vi "test_Error Code Channel_Overwrite File If Exists Disabled.vi"(8 "error in (no error)":errorcluster, 11 "TestCase in":refnum<class "Telemetry System Tests.lvclass">=refnum) -> (0 "error out":errorcluster, 3 "TestCase out":refnum<class "Telemetry System Tests.lvclass">)   [LabVIEW 2026, in "Telemetry System Tests.lvclass"]
uses:
  Telemetry System Tests.lvclass
  b15e678b-00b4-460c-84a3-511904b6b81c.vi
  <vilib>/NI VeriStand/Execution/Workspace/NI_VS Workspace ExecutionAPI.lvlib
  Telemetry Test Utilities/Telemetry Test Utilities.lvlib
  b783cf42-fd76-406f-8202-c013ab39f902.vi
  0f18a7fd-8127-48b0-8de3-31218f8e8d95.vi
  addb9b33-6ae5-4271-aa15-5e9a5667d6da.vi
  <vilib>/NI VeriStand/Execution/Workspace/NI VeriStand - Get Single Channel Value.vi
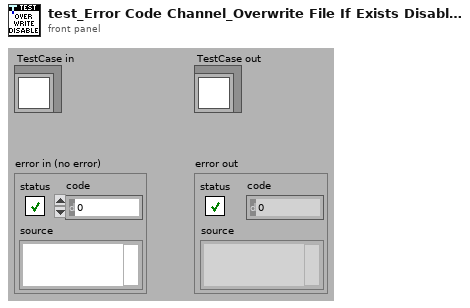
[diagram p1: front panel]
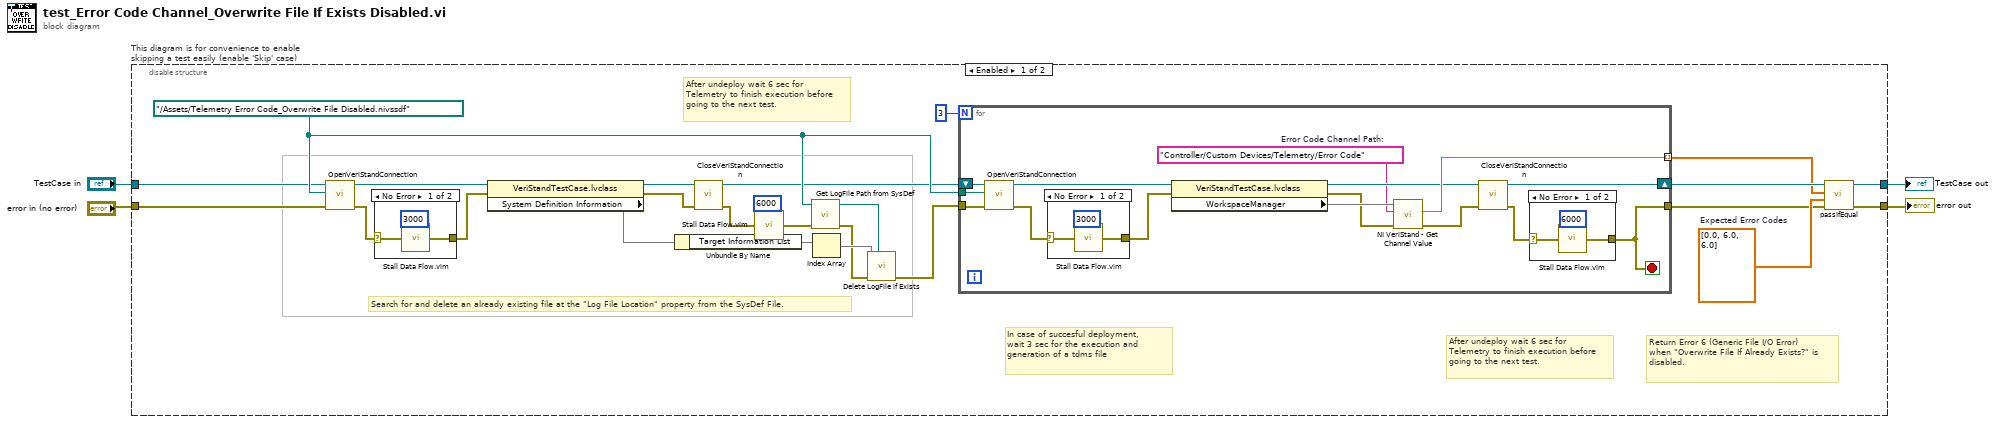
[diagram p0: block diagram]
diagram:
  n1 = disable-structure "This diagram is for convenience to enable skipping a test easily (enable 'Skip' case)" shown="Enabled" {
    disable-tunnel: "TestCase in" -> [w15 w60]
    disable-tunnel: [w23 w58] -> w1
    disable-tunnel: [w24 w59] -> w3
    disable-tunnel: "error in (no error)" -> [w18 w57]
    frame Enabled {
      w26 = dbl[] [0.0, 6.0, 6.0]  # Expected Error Codes
      w16 = path "../Assets/Telemetry Error Code_Overwrite File Disabled.nivssdf" ("System Definition File")
      # "In case of succesful deployment, wait 3 sec for the execution and generation of a tdms file"
      # "After undeploy wait 6 sec for Telemetry to finish execution before going to the next test."
      # "After undeploy wait 6 sec for Telemetry to finish execution before going to the next test."
      # "Search for and delete an already existing file at the \"Log File Location\" property from the SysDef File."
      # "Return Error 6 (Generic File I/O Error) when \"Overwrite File If Already Exists?\" is disabled."
      n2 = call-dynamic "OpenVeriStandConnection.vi"("error in (no error)"=w18, "System Definition File"=w16, "VeriStand Test Case in"=w15) -> ("error out"=w17:errorcluster, "VeriStand Test Case out"=w14:refnum<class "VeriStandTestCase.lvclass">)  [unwired: 6 in, 1 out]
      n3 = case shown="No Error" w17 {
        selector: w17 -> [w32 w33]
        tunnel: [w30 w33] -> w10
        frame No Error {
          n4 = call "Stall Data Flow.vim"("value in"=w32, "milliseconds to wait"=u32 3000) -> ("value out"=w30:errorcluster)  [unwired: 1 out]
        }
        frame Error {
        }
      }
      n5 = property class="VeriStandTestCase.lvclass"(reference=w14, error in=w10) -> (reference out=w13:refnum<class "VeriStandTestCase.lvclass">, error out=w12:errorcluster, "System Definition Information"=w11)
      n6 = Unbundle By Name(w11) -> ("Target Information List"=w20)
      n7 = call-dynamic "CloseVeriStandConnection.vi"("error in (no error)"=w12, "VeriStand Test Case in"=w13) -> ("error out"=w8:errorcluster, "VeriStand Test Case out"=w9:refnum<class "VeriStandTestCase.lvclass">)  [unwired: 8 in]
      n8 = call "Stall Data Flow.vim"("value in"=w8, "milliseconds to wait"=u32 6000) -> ("value out"=w6:errorcluster)  [unwired: 1 out]
      n9 = call "Get LogFile Path from SysDef.vi"("error in (no error)"=w6, "System Definition File"=w16) -> ("error out"=w7:errorcluster, "Log File Path"=w22:path)  [unwired: 8 in]
      n10 = Index Array(array=w20) -> (element=w19)  [unwired: 1 in]
      n11 = call "Delete LogFile if Exists.vi"("Log File Path"=w22, "error in (no error)"=w7, "Target Information"=w19) -> ("error out"=w21:errorcluster)  [unwired: 8 in]
      n12 = for {
        N: 3 -> [_]
        tunnel: w21 -> [w48]
        tunnel: w16 -> [w45]
        shift-right: [w44] -> w29
        shift-left: w9 -> [w46]
        tunnel: [w42] -> w27 mode=indexing
        tunnel: [w35] -> w25
        stop <- w35 stop-if-true
        w37 = "Controller/Custom Devices/Telemetry/Error Code"  # Error Code Channel Path:
        n13 = call-dynamic "OpenVeriStandConnection.vi"("error in (no error)"=w48, "System Definition File"=w45, "VeriStand Test Case in"=w46) -> ("error out"=w47:errorcluster, "VeriStand Test Case out"=w36:refnum<class "VeriStandTestCase.lvclass">)  [unwired: 6 in, 1 out]
        n14 = case shown="No Error" w47 {
          selector: w47 -> [w55 w56]
          tunnel: [w53 w56] -> w41
          frame No Error {
            n15 = call "Stall Data Flow.vim"("value in"=w55, "milliseconds to wait"=u32 3000) -> ("value out"=w53:errorcluster)  [unwired: 1 out]
          }
          frame Error {
          }
        }
        n16 = property class="VeriStandTestCase.lvclass"(reference=w36, error in=w41) -> (reference out=w40:refnum<class "VeriStandTestCase.lvclass">, error out=w38:errorcluster, "WorkspaceManager"=w39)
        n17 = call-poly <vilib>:"NI VeriStand - Get Channel Value.vi"("error in (no error)"=w38, "Channel"=w37, "WorkspaceManager in"=w39) -> ("error out"=w43:errorcluster, "Value"=w42:dbl)  [unwired: 6 in, 1 out]
        n18 = call-dynamic "CloseVeriStandConnection.vi"("error in (no error)"=w43, "VeriStand Test Case in"=w40) -> ("error out"=w34:errorcluster, "VeriStand Test Case out"=w44:refnum<class "VeriStandTestCase.lvclass">)  [unwired: 8 in]
        n19 = case shown="No Error" w34 {
          selector: w34 -> [w49 w52]
          tunnel: [w51 w52] -> w35
          frame No Error {
            n20 = call "Stall Data Flow.vim"("value in"=w49, "milliseconds to wait"=u32 6000) -> ("value out"=w51:errorcluster)  [unwired: 1 out]
          }
          frame Error {
          }
        }
      }
      n21 = call-dynamic "passIfEqual.vi"("error in (no error)"=w25, "y"=w26, "x"=w27, "TestCase in"=w29) -> ("error out"=w24:errorcluster, "TestCase out"=w23:refnum<class "Telemetry System Tests.lvclass">)  [unwired: 6 in]
    }
    frame Disabled {
      # "skip test result while test is under development"
      n22 = call <vilib>:"skip.vi"("error in (no error)"=w57, "TestCase in"=w60) -> ("error out"=w59:errorcluster, "TestCase out"=w58:refnum<class "Telemetry System Tests.lvclass">)  [unwired: 8 in]
    }
  }
  "error out" <- w3
  "TestCase out" <- w1
